vi "Configure Output Couple.vi"(8 "error in (no error)":errorcluster, 9 "Couple Delay Offset (0 s)":dbl, 10 "Enable Output Couple (F: Disable)":bool, 11 "VISA resource name":refnum<visa-resource-name>) -> (0 "error out":errorcluster, 3 "VISA resource name out":refnum<visa-resource-name>)   [LabVIEW 2021, in "Agilent N6900 N7900 Series.lvlib"]
doc: "Enables or disables output coupling. Output coupling allows the outputs of multiple instruments to turn on and off sequentially.\n\nNote: The values that are set are persistant through a reset. Thus, it may be wise to always set this VI to the desired values."
uses:
  <instrlib>/Agilent N6900 N7900 Series/Agilent N6900 N7900 Series.lvlib
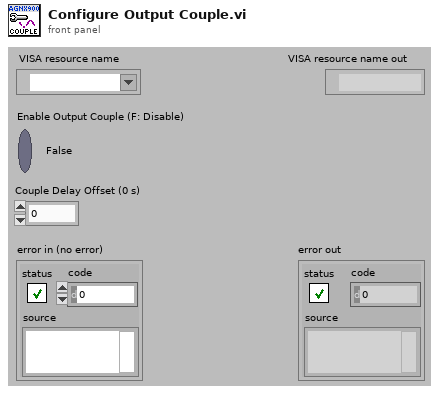
[diagram p1: front panel]
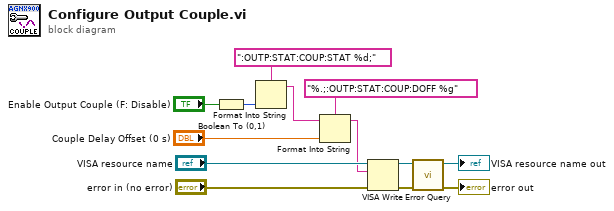
[diagram p0: block diagram]
diagram:
  n1 = Boolean To (0,1)(Boolean="Enable Output Couple (F: Disable)") -> (0, 1=w3:i16)
  n2 = Format Into String(format string=":OUTP:STAT:COUP:STAT %d;", w3) -> (resulting string=w4:string)  [unwired: 2 in, 1 out]
  n3 = Format Into String(format string="%.;:OUTP:STAT:COUP:DOFF %g", initial string=w4, "Couple Delay Offset (0 s)") -> (resulting string=w5:string)  [unwired: 1 in, 1 out]
  n4 = VISA Write(VISA resource name="VISA resource name", write buffer=w5, error in (no error)="error in (no error)") -> (VISA resource name out=w10:refnum<visa-resource-name>, error out=w11:errorcluster)  [unwired: 1 out]
  n5 = call <instrlib>:"Error Query.vi"("error in (no error)"=w11, "VISA resource name"=w10) -> ("error out"=→"error out":errorcluster, "VISA resource name out"=→"VISA resource name out":refnum<visa-resource-name>)  [unwired: 6 in, 2 out]
